vi "Chunck to paragraph.vi"(7 "Leading":sgl=1.5, 8 "error in (no error)":errorcluster, 9 "Font":refnum<k24>, 10 "Hyperlink":T1) -> (0 "error out":errorcluster, 2 "Anchor":refnum<k24>)   [LabVIEW 2012]
doc: "Creates a <B>text hyperlink</B>.\n\nVersion 1.0\nDeveloped by Jean-Marc Simard\nCopyright © 2010, Exaprom Inc.\nAll rights reserved.\nLicense: BSD\n\nWith iTextSharp 4.1.6 (http://itextsharp.sourceforge.net)\nunder Mozilla Public License Version 1.1\n(http://www.mozilla.org/MPL/MPL-1.1.html)"
uses:
  C:/Users/MaxCorp/Documents/GitHub/TopView/DLL/itextsharp.dll
  GitHub/TopView/DLL/itextsharp.dll
  Controls/Text and Hypertext.ctl
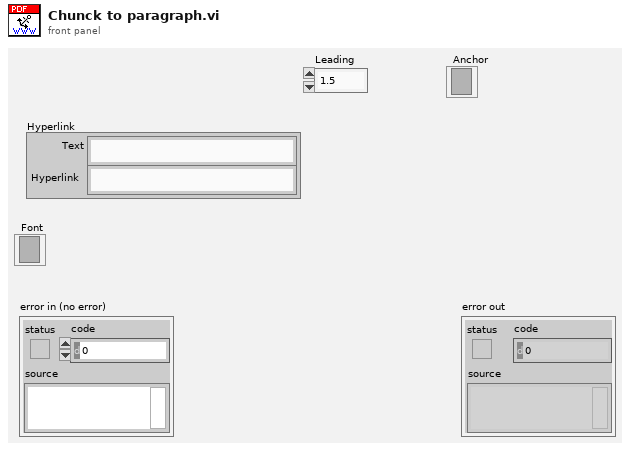
[diagram p1: front panel]
types:
  T1 = typedef "Text and Hypertext.ctl" = cluster{"Text":string, "Hyperlink":string}
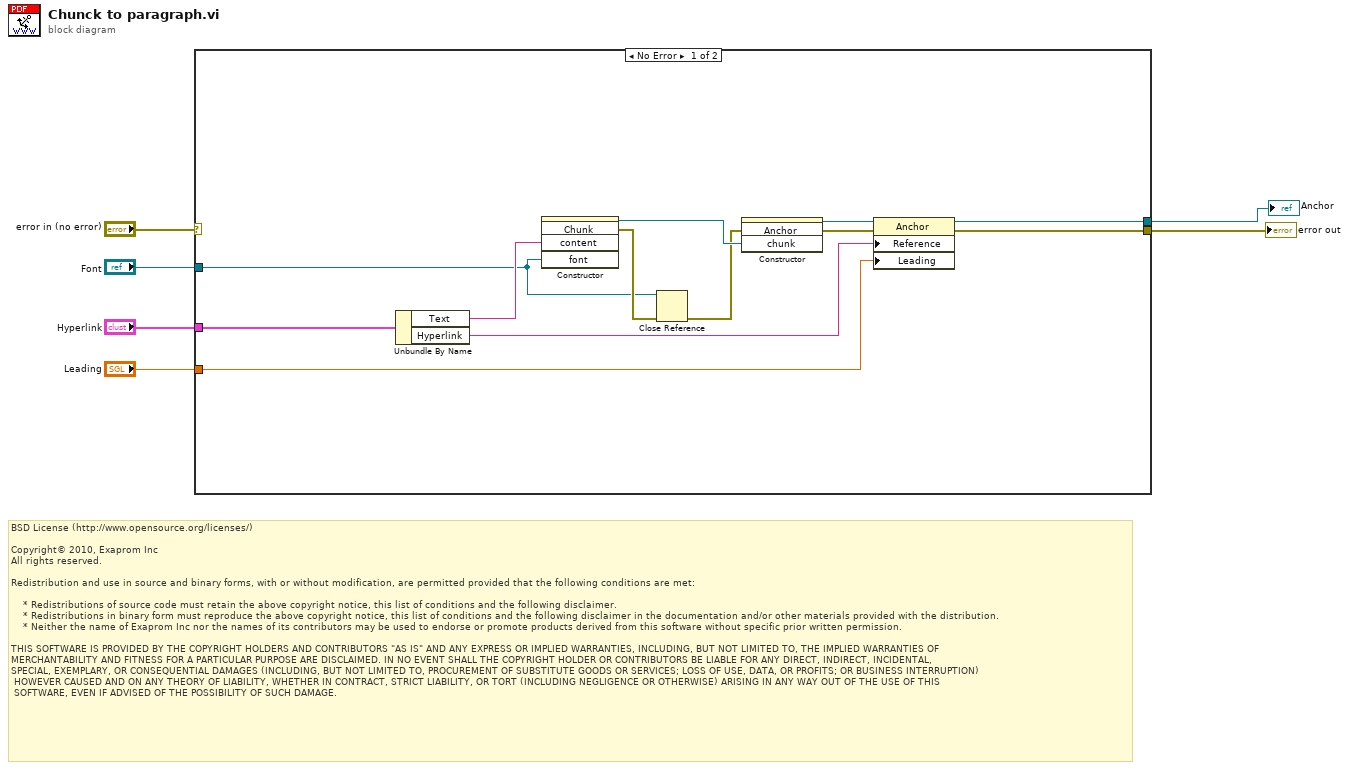
[diagram p0: block diagram]
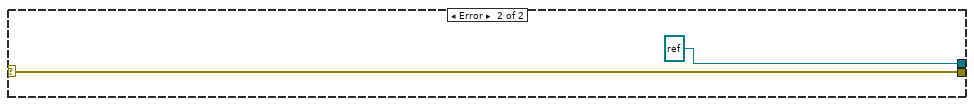
[diagram p2: hidden frame]
diagram:
  # "BSD License (http://www.opensource.org/licenses/)\n\nCopyright© 2010, Exaprom Inc\nAll rights reserved.\n\nRedistribution and use in source and binary forms, with or without modification, are permitted provided that the following conditions are met:\n\n    * Redistributions of source code must retain the above copyright notice, this list of conditions and the following disclaimer.\n    * Redistributions in binary form must reproduce the above copyright notice, this list of conditions and the following disclaimer in the documentation and/or other materials provided with the distribution.\n    * Neither the name of Exaprom Inc nor the names of its contributors may be used to endorse or promote products derived from this software without specific prior written permission.\n\nTHIS SOFTWARE IS PROVIDED BY THE COPYRIGHT HOLDERS AND CONTRIBUTORS \"AS IS\" AND ANY EXPRESS OR IMPLIED WARRANTIES, INCLUDING, BUT NOT LIMITED TO, THE IMPLIED WARRANTIES OF \nMERCHANTABILITY AND FITNESS FOR A PARTICULAR PURPOSE ARE DISCLAIMED. IN NO EVENT SHALL THE COPYRIGHT HOLDER OR CONTRIBUTORS BE LIABLE FOR ANY DIRECT, INDIRECT, INCIDENTAL,\nSPECIAL, EXEMPLARY, OR CONSEQUENTIAL DAMAGES (INCLUDING, BUT NOT LIMITED TO, PROCUREMENT OF SUBSTITUTE GOODS OR SERVICES; LOSS OF USE, DATA, OR PROFITS; OR BUSINESS INTERRUPTION)\n HOWEVER CAUSED AND ON ANY THEORY OF LIABILITY, WHETHER IN CONTRACT, STRICT LIABILITY, OR TORT (INCLUDING NEGLIGENCE OR OTHERWISE) ARISING IN ANY WAY OUT OF THE USE OF THIS\n SOFTWARE, EVEN IF ADVISED OF THE POSSIBILITY OF SUCH DAMAGE."
  n1 = case shown="No Error" "error in (no error)" {
    selector: "error in (no error)" -> [_ w20]
    tunnel: [w12 w20] -> w6
    tunnel: "Hyperlink" -> [w18 _]
    tunnel: [w11 refnum<k24> refnum ("hidden reference")] -> w3
    tunnel: "Leading" -> [w8 _]
    tunnel: "Font" -> [w7 _]
    frame No Error {
      n2 = Unbundle By Name(w18) -> ("Text"=w13:string, "Hyperlink"=w17:string)
      n3 = constructor class="Chunk"("content"=w13, "font"=w7) -> (reference out=w14:refnum<k24>, error out=w10:errorcluster)  [unwired: 3 in, 3 out]
      n4 = Close Reference(reference=w7, error in (no error)=w10) -> (error out=w9:errorcluster)
      n5 = constructor class="Anchor"(error in=w9, "chunk"=w14) -> (reference out=w15:refnum<k24>, error out=w16:errorcluster)  [unwired: 2 in, 2 out]
      n6 = property class="Anchor"(reference=w15, error in=w16, "Reference"=w17, "Leading"=w8) -> (reference out=w11:refnum<k24>, error out=w12:errorcluster)
    }
    frame Error {
    }
  }
  "error out" <- w6
  "Anchor" <- w3
